vi "test_read_analog_worker.vi"() -> ()   [LabVIEW 2017]
uses:
  support/Message Queue/Enqueue Message (Single).vi
  <vilib>/Utility/error.llb/Error Cluster From Error Code.vi
  <vilib>/ErrorRing/Error Ring.xnode
  measurement_result/MeasurementResult.lvclass
  support/Message Queue/Message Queue.lvlib
  support/User Event - Stop/User Event - Stop.lvlib
  logger/logger.lvlib
panel:
  out "raw_data":u16[][](array[numeric])
  in  "change hardware":bool
  in  "stop":bool
  in  "Play Button":bool
  out "status":string
  in  "Exit":bool
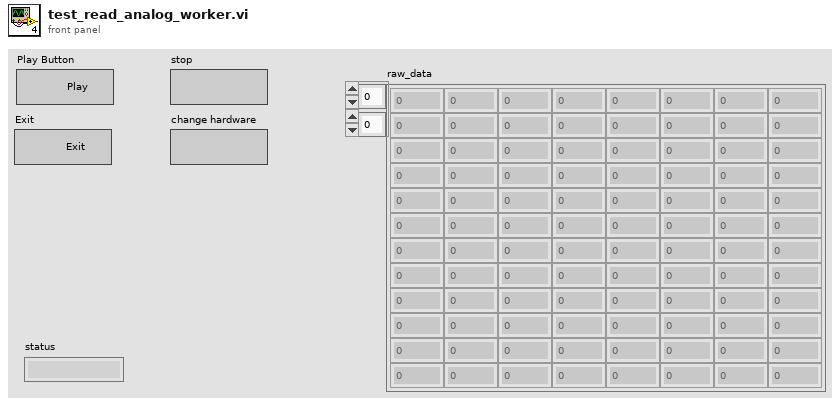
[diagram p1: front panel]
types:
  T1 = typedef "Message Queue.lvlib/All Message Queues.ctl" = cluster{"MHL":refnum<queue>, "TCPServerLoop":refnum<queue>, "RequestProcessorLoop":refnum<queue>, "AnalogReadWorkerLoop":refnum<queue>, "AnalogWriteWorkerLoop":refnum<queue>, "DigitalReadWorkerLoop":refnum<queue>, "DigitalWriteWorkerLoop":refnum<queue>}
  T2 = typedef "Notifiers.ctl" = cluster{"TCPServerExit":refnum<notifier>, "RequestProcesscorExit":refnum<notifier>, "AnalogReadWorkerrExit":refnum<notifier>, "AnalogWriteWorkerrExit":refnum<notifier>, "DigitalReadWorkerrExit":refnum<notifier>, "DigitalWriteWorkerrExit":refnum<notifier>}
  T3 = typedef "data_Notifiers.ctl" = cluster{"AnalogMeasurementResult":refnum<notifier>}
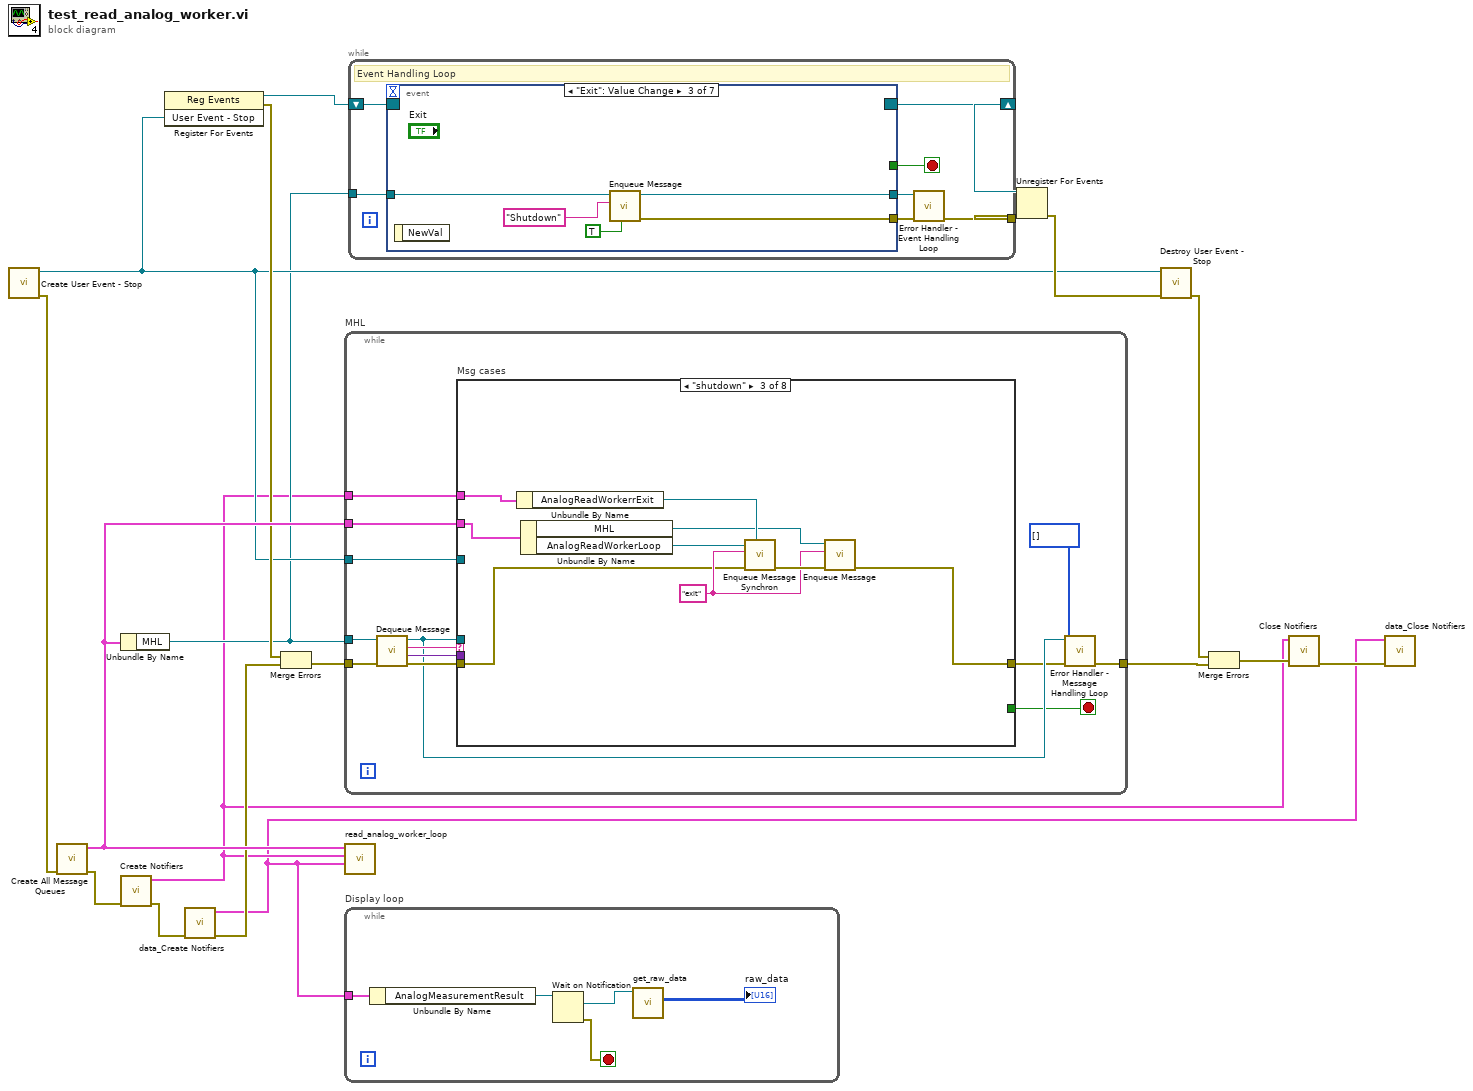
[diagram p0: block diagram]
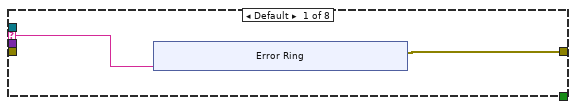
[diagram p2: hidden frame]
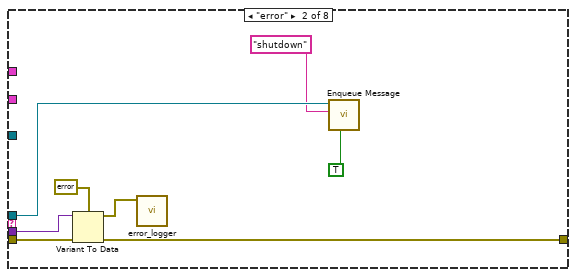
[diagram p3: hidden frame]
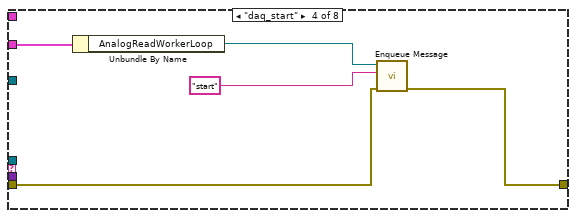
[diagram p4: hidden frame]
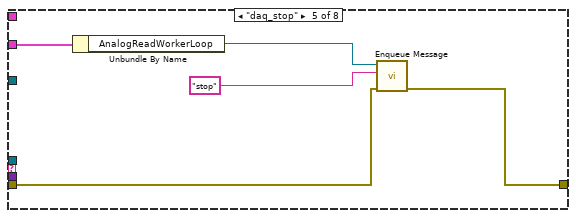
[diagram p5: hidden frame]
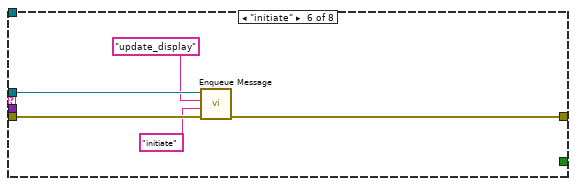
[diagram p6: hidden frame]
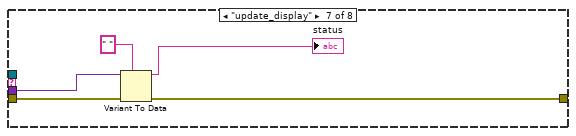
[diagram p7: hidden frame]
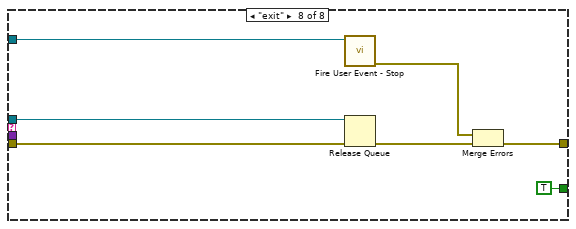
[diagram p8: hidden frame]
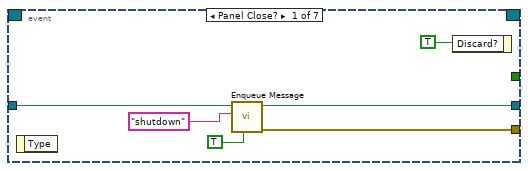
[diagram p9: hidden frame]
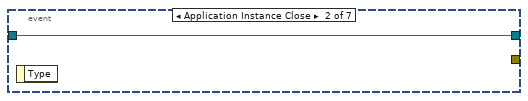
[diagram p10: hidden frame]
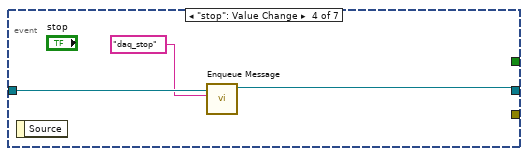
[diagram p11: hidden frame]
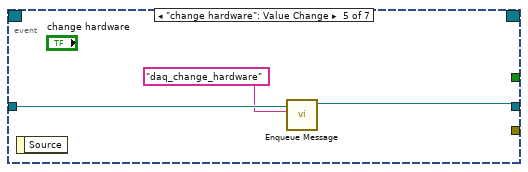
[diagram p12: hidden frame]
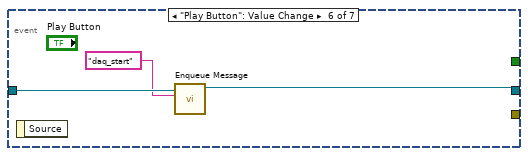
[diagram p13: hidden frame]
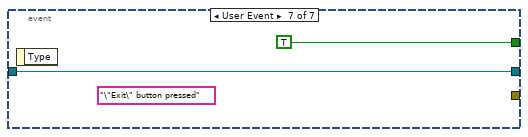
[diagram p14: hidden frame]
diagram:
  n1 = call "Create User Event - Stop.vi"() -> ("error out"=w14:errorcluster, "User Event - Stop"=w8:refnum<user-event>)  [unwired: 10 in]
  n2 = call "Create All Message Queues.vi"("error in (no error)"=w14) -> ("error out"=w13:errorcluster, "Message Queues out"=w15:T1)  [unwired: 9 in]
  n3 = Unbundle By Name(w15) -> ("MHL"=w7:refnum<queue>)
  n4 = call "Create Notifiers.vi"("error in"=w13) -> ("error out"=w12:errorcluster, "Notifiers"=w2:T2)  [unwired: 9 in]
  n5 = register-events(w8) -> (reference out=w18:refnum<event-registration>, error out=w10:errorcluster)  [unwired: 2 in]
  n6 = call "data_Create Notifiers.vi"("error in"=w12) -> ("error out"=w9:errorcluster, "output cluster"=w1:T3)  [unwired: 9 in]
  n7 = Merge Errors(w10, w9) -> (w11:errorcluster)
  n8 = while "MHL" {
    tunnel: w11 -> [w29]
    tunnel: w7 -> [w28]
    tunnel: w15 -> [w27]
    tunnel: w8 -> [w26]
    tunnel: w2 -> [w22]
    tunnel: [w21] -> w4
    stop <- w23 stop-if-true
    n9 = call "Dequeue Message.vi"("error in (no error)"=w29, "Message Queue"=w28) -> ("error out"=w30:errorcluster, "Message Data"=w31:variant, "Message"=w32:string, "dup Message Queue"=w25:refnum<queue>)  [unwired: 6 in]
    n10 = case "Msg cases" shown="\"shutdown\"" w32 {
      selector: w32 -> [w34 _ _ _ _ _ _ _]
      tunnel: w25 -> [_ w49 _ _ _ w70 _ w83]
      tunnel: w31 -> [_ w44 _ _ _ _ w76 _]
      tunnel: w30 -> [_ w43 w50 w59 w64 w73 w78 w84]
      tunnel: w27 -> [_ _ w56 w63 w68 _ _ _]
      tunnel: w26 -> [_ _ _ _ _ _ _ w82]
      tunnel: [w33 w42 w51 w60 w65 w72 w77 w79] -> w24
      tunnel: [_ _ _ _ _ _ _ TRUE] -> w23
      tunnel: w22 -> [_ _ w58 _ _ _ _ _]
      frame Default {
        n11 = xnode "Error Ring"("parameter 0"=w34) -> ("error out"=w33:errorcluster)
      }
      frame "error" {
        n12 = Variant To Data(error in=w43, type=errorcluster {"status"=FALSE, "code"=0, "source"=""} ("error constant"), Variant=w44) -> (data=w45:errorcluster, error out=w42:errorcluster)
        n13 = call "error_logger.vi"("error in (no error)"=w45) -> ()  [unwired: 11 in]
        n14 = call-poly "Enqueue Message.vi"("Priority Message? (F)"=TRUE, "Message"="shutdown", "Message Queue"=w49) -> ()  [unwired: 7 in, 2 out]
      }
      frame "shutdown" {
        w52 = "exit"
        n15 = Unbundle By Name(w58) -> ("AnalogReadWorkerrExit"=w57:refnum<notifier>)
        n16 = Unbundle By Name(w56) -> ("MHL"=w54:refnum<queue>, "AnalogReadWorkerLoop"=w55:refnum<queue>)
        n17 = call "Enqueue Message Synchron.vi"("Notifier"=w57, "error in (no error)"=w50, "Message"=w52, "Message Queue"=w55) -> ("error out"=w53:errorcluster)  [unwired: 6 in, 1 out]
        n18 = call-poly "Enqueue Message.vi"("error in (no error)"=w53, "Message"=w52, "Message Queue"=w54) -> ("error out"=w51:errorcluster)  [unwired: 7 in, 1 out]
      }
      frame "daq_start" {
        n19 = Unbundle By Name(w63) -> ("AnalogReadWorkerLoop"=w62:refnum<queue>)
        n20 = call-poly "Enqueue Message.vi"("error in (no error)"=w59, "Message"="start", "Message Queue"=w62) -> ("error out"=w60:errorcluster)  [unwired: 7 in, 1 out]
      }
      frame "daq_stop" {
        n21 = Unbundle By Name(w68) -> ("AnalogReadWorkerLoop"=w67:refnum<queue>)
        n22 = call-poly "Enqueue Message.vi"("error in (no error)"=w64, "Message"="stop", "Message Queue"=w67) -> ("error out"=w65:errorcluster)  [unwired: 7 in, 1 out]
      }
      frame "initiate" {
        n23 = call-poly "Enqueue Message.vi"("error in (no error)"=w73, "Message Data"="initiate" ("status"), "Message"="update_display", "Message Queue"=w70) -> ("error out"=w72:errorcluster)  [unwired: 6 in, 1 out]
      }
      frame "update_display" {
        n24 = Variant To Data(error in=w78, type=" ", Variant=w76) -> (data=→"status":string, error out=w77:errorcluster)
      }
      frame "exit" {
        n25 = call "Fire User Event - Stop.vi"("User Event - Stop"=w82) -> ("error out"=w81:errorcluster)  [unwired: 10 in]
        n26 = Release Queue(queue=w83, error in (no error)=w84) -> (error out=w80:errorcluster)  [unwired: 1 in, 2 out]
        n27 = Merge Errors(w81, w80) -> (w79:errorcluster)
      }
    }
    n28 = call "Error Handler - Message Handling Loop.vi"("error in (no error)"=w24, "Ignore Errors (Runtime)"=i32[] [], "Message Queue"=w25) -> ("dup error in"=w21:errorcluster)  [unwired: 7 in, 1 out]
  }
  n29 = call "read_analog_worker_loop.vi"("Data Notifiers"=w1, "Notifiers"=w2, "Message Queues"=w15) -> ()  [unwired: 8 in, 1 out]
  n30 = while "Display loop" {
    tunnel: w1 -> [w90]
    stop <- w88 stop-if-true
    n31 = Unbundle By Name(w90) -> ("AnalogMeasurementResult"=w89:refnum<notifier>)
    n32 = Wait on Notification(notifier=w89) -> (notification=w87:refnum<class "MeasurementResult.lvclass">, error out=w88:errorcluster)  [unwired: 3 in, 2 out]
    n33 = call-dynamic "get_raw_data.vi"("MeasurementResult in"=w87) -> ("raw_data"=→"raw_data":u16[][])  [unwired: 8 in, 2 out]
  }
  n34 = while {
    shift-right: [w92] -> w16
    shift-left: w18 -> [w93]
    tunnel: [w94] -> w19
    tunnel: w7 -> [w91]
    stop <- w96 stop-if-true
    # "Event Handling Loop"
    n35 = event shown="[2] \"Exit\": Value Change" {
      selector: w93 -> [_ _ _ _ _ _ _]
      dyn-events: [_ _ _ _ _ _ _] -> w92
      timeout: _ -> [_ _ _ _ _ _ _]
      tunnel: [_ _ _ _ _ _ TRUE ("Discard?")] -> w96
      tunnel: [w102 _ w109 _ _ _ _] -> w97
      tunnel: [w101 w104 w108 w111 w114 w116 w119] -> w95
      tunnel: w91 -> [w98 w104 w105 w112 w115 w118 w119]
      event Panel Close? {
        n36 = event-data() -> ()  [unwired: 1 in, 1 out]
        n37 = call-poly "Enqueue Message.vi"("Priority Message? (F)"=TRUE, "Message"="shutdown", "Message Queue"=w98) -> ("error out"=w102:errorcluster, "dup Message Queue"=w101:refnum<queue>)  [unwired: 7 in]
        n38 = event-data("Discard?"=TRUE) -> ()  [unwired: 1 in, 1 out]
      }
      event Application Instance Close {
        n39 = event-data() -> ()  [unwired: 1 in, 1 out]
      }
      event "Exit": Value Change {
        n40 = event-data() -> ()  [unwired: 1 in, 1 out]
        n41 = call-poly "Enqueue Message.vi"("Priority Message? (F)"=TRUE, "Message"="Shutdown", "Message Queue"=w105) -> ("error out"=w109:errorcluster, "dup Message Queue"=w108:refnum<queue>)  [unwired: 7 in]
      }
      event "stop": Value Change {
        n42 = event-data() -> ()  [unwired: 1 in, 1 out]
        n43 = call-poly "Enqueue Message.vi"("Message"="daq_stop", "Message Queue"=w112) -> ("dup Message Queue"=w111:refnum<queue>)  [unwired: 8 in, 1 out]
      }
      event "change hardware": Value Change {
        n44 = event-data() -> ()  [unwired: 1 in, 1 out]
        n45 = call-poly "Enqueue Message.vi"("Message"="daq_change_hardware", "Message Queue"=w115) -> ("dup Message Queue"=w114:refnum<queue>)  [unwired: 8 in, 1 out]
      }
      event "Play Button": Value Change {
        n46 = event-data() -> ()  [unwired: 1 in, 1 out]
        n47 = call-poly "Enqueue Message.vi"("Message"="daq_start", "Message Queue"=w118) -> ("dup Message Queue"=w116:refnum<queue>)  [unwired: 8 in, 1 out]
      }
      event User Event {
        (unwired) "\"Exit\" button pressed" ("VI Stopped")
        n48 = event-data() -> ()  [unwired: 1 in, 1 out]
      }
    }
    n49 = call "Error Handler - Event Handling Loop.vi"("error in (no error)"=w97, "Message Queue"=w95) -> ("dup error in"=w94:errorcluster)  [unwired: 8 in, 1 out]
  }
  n50 = Unregister For Events(event registration refnum=w16, error in=w19) -> (error out=w17:errorcluster)
  n51 = call "Destroy User Event - Stop.vi"("error in (no error)"=w17, "User Event - Stop"=w8) -> ("error out"=w5:errorcluster)  [unwired: 9 in]
  n52 = Merge Errors(w5, w4) -> (w3:errorcluster)
  n53 = call "Close Notifiers.vi"("error in"=w3, "Notifiers"=w2) -> ("error out"=w6:errorcluster)  [unwired: 9 in]
  n54 = call "data_Close Notifiers.vi"("error in"=w6, "Data Notifiers"=w1) -> ()  [unwired: 9 in, 1 out]
